vi "Write Data.vi"(8 "error in (no error)":errorcluster, 9 "Publication Time":timestamp, 10 "Value":variant, 11 "EventTransport In":refnum<class "EventTransport.lvclass">) -> (0 "error out":errorcluster, 3 "EventTransport Out":refnum<class "EventTransport.lvclass">)   [LabVIEW 2015, in "Mediator.lvlib" / "EventTransport.lvclass"]
doc: "<License>\nCopyright © 2017 Composed Systems, LLC | All rights reserved\nwww.composed.io\n\nAuthor: Ethan Stern <ethan.stern@composed.io>\n\nThis software is provided \"AS IS\" WITHOUT WARRANTIES, either express or implied, AND IS FOR EDUCATIONAL PURPOSES ONLY.\n</License>"
uses:
  EventTransport.lvclass
  EventTransport.lvclass/EventTransport.ctl
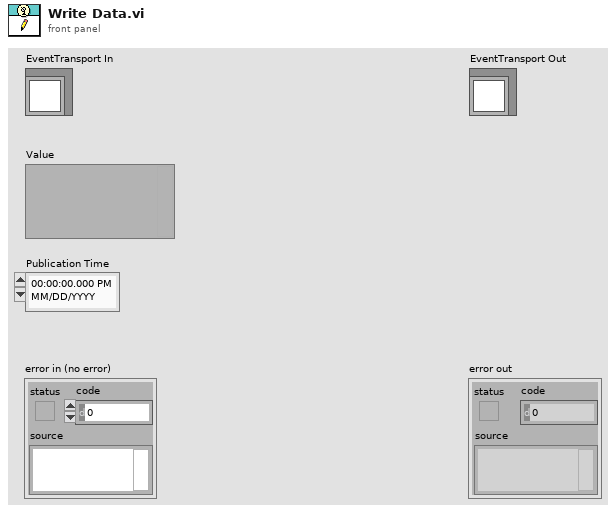
[diagram p1: front panel]
types:
  T1 = typedef "usereventprio.ctl" = enum32{"high priority", "normal priority"}
  T2 = cluster{"Value":variant, "Publication Time":timestamp}
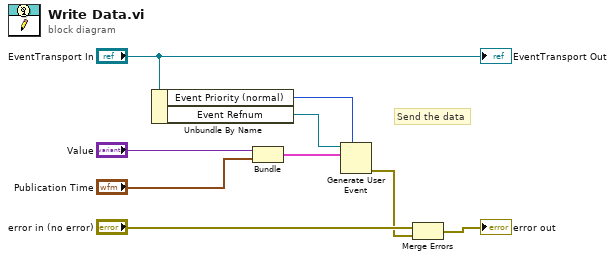
[diagram p0: block diagram]
diagram:
  # "Send the data"
  n1 = Unbundle By Name("EventTransport In") -> ("Event Priority (normal)"=w1:T1, "Event Refnum"=w8:refnum<user-event>)
  n2 = Bundle("Value"="Value", "Publication Time"="Publication Time") -> (w2:T2)  [unwired: 1 in]
  n3 = Generate User Event(priority (normal)=w1, user event=w8, event data cluster=w2) -> (error out=w5:errorcluster)  [unwired: 1 in, 1 out]
  n4 = Merge Errors("error in (no error)", w5) -> (→"error out":errorcluster)
  "EventTransport Out" <- "EventTransport In"
